vi "Na-DAS_7609 Single.vi"(1 "Single Na-Das Device":T1) -> (0 "DAQ Error":errorcluster)   [LabVIEW 2021]
doc: "Use this plug-in with the Nathan 7609 data acquisition system"
uses:
  Device ID port info.ctl
  Sub_vis/Upload Data.ctl
  Globals/Meas_global.vi
  Globals/Extra_Commands_Global.vi
  Globals/Trav_pos_global.vi
  Globals/Dynamic_call_global.ph.vi
panel:
  in  "Minimum timeout (ms)":u32=15000
  in  "Input voltage range (V)":u8(ring)=1 items=["-5... +5 V", "-10... +10 V"]
  out "Config read-back ok":bool
  out "Overruns":u32
  # "Do not close this window between blocks"
  # "PN 25/11/2014, 19/12/2014, 15/02/2015 (channels in any order), 17/08/2015 (stop ack mod), 23/08/2015 (timeout mod for SW vs HW triggering), 03/09/2017 (rising and falling edge options for HW triggering), 06/06/2018 (rendezvous),"
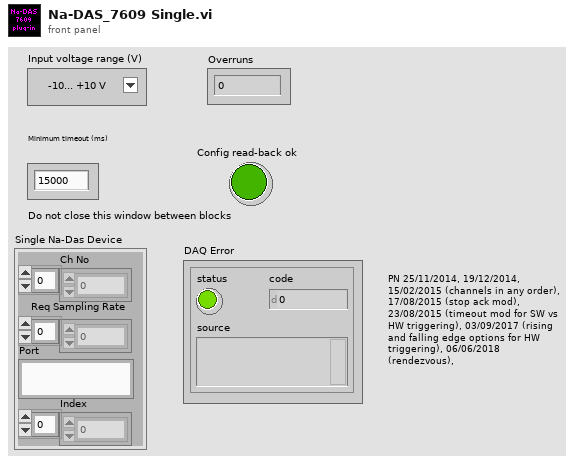
[diagram p1: front panel]
types:
  T1 = typedef "Device ID port info.ctl" = cluster{"Ch No":i16[], "Req Sampling Rate":dbl[], "Port":string, "Index":i32[]}
  T2 = typedef "Traverse_cluster.ctl" = cluster{"Start X":sgl, "Start Y":sgl, "Start Z":sgl, "End X":sgl, "End Y":sgl, "End Z":sgl, "nPoints":i32, "Spacing":T3, "Filename":path, "Tunnel Speed":dbl, "Averaging time (mins)":dbl, "Extra Commands":string, "Carrier_1 Q (l/min)":dbl, "Carrier_2 Q (l/min)":dbl, "Trace Gas Concentration (%)":dbl, "Specific Arguments":string, "Comments":string, "Row No":i32, "Row Type Selector":T4, "EstCompl":string, "Row Duration (mins)":dbl, "nValidPoints":i32, "Meas Setup File":string}
  T3 = typedef "Spacing.ctl" = enum16{"Linear", "Log", "Gauss", "Specified", "N/A"}
  T4 = typedef "Multi_run_mode.ctl" = enum16{"Move Traverse Only", "Set Tunnel Speed Only", "Set Source Only", "Set Measurement Conditions", "Single Measurement", "Vertical Profile", "Lateral Profile", "Longitudinal Profile", "Multi-Axis Profile", "Explore Volume", "Auto Calibrate", "Meas Fast FID Bkgnd", "Check Beam Power", "Scanning Valve Measurement", "Run VI Named:", "Set ADAM Ch", "Wait (minutes)", "Send Message", "Synchronize With:", "Fall Back to this Row", "Turn Off Row Repeating", "Traverse 3D Volume", "Blank Row", "Jump to Fall Back Row"}
  T5 = typedef "Trigger_Mode.ctl" = enum16{"Free Running", "Start on Trigger", "Trigger Every Block", "Trigger Every Sample"}
  T6 = typedef "Setup.ctl" = enum16{"Run Program", "Show Setup", "Save Current Setup", "Setup Front Panel"}
  T7 = typedef "Upload Data.ctl" = enum16{"Voltage Array", "Time Trace Cluster"}
  T8 = typedef "NA-Das_7609.ctl" = cluster{"Timeout (ms)":u32, "N channels bytes to read":u8, "Triggering mode":u8, "Input voltage range (V)":u8, "Oversampling ratio":u8}
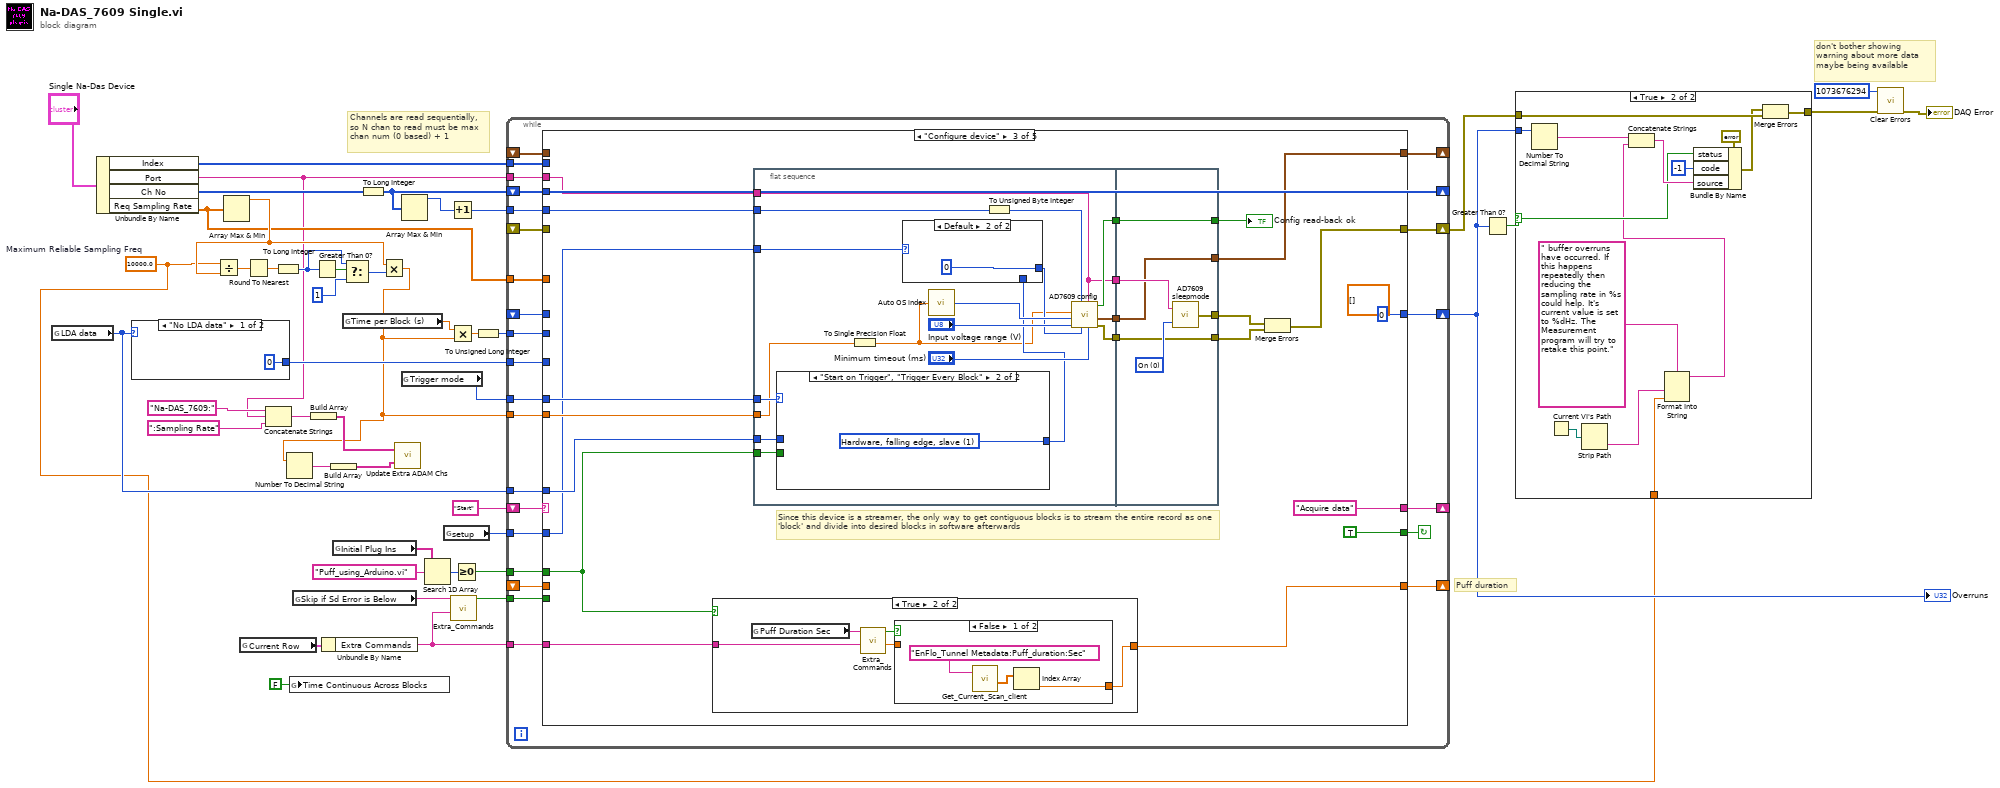
[diagram p0: block diagram]
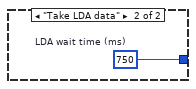
[diagram p3: hidden frame]
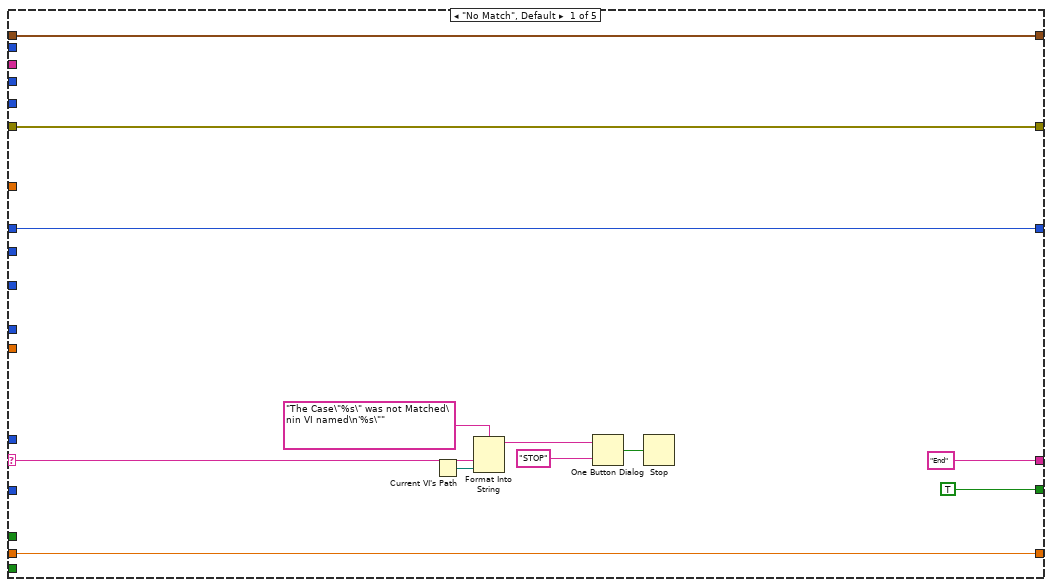
[diagram p4: hidden frame]
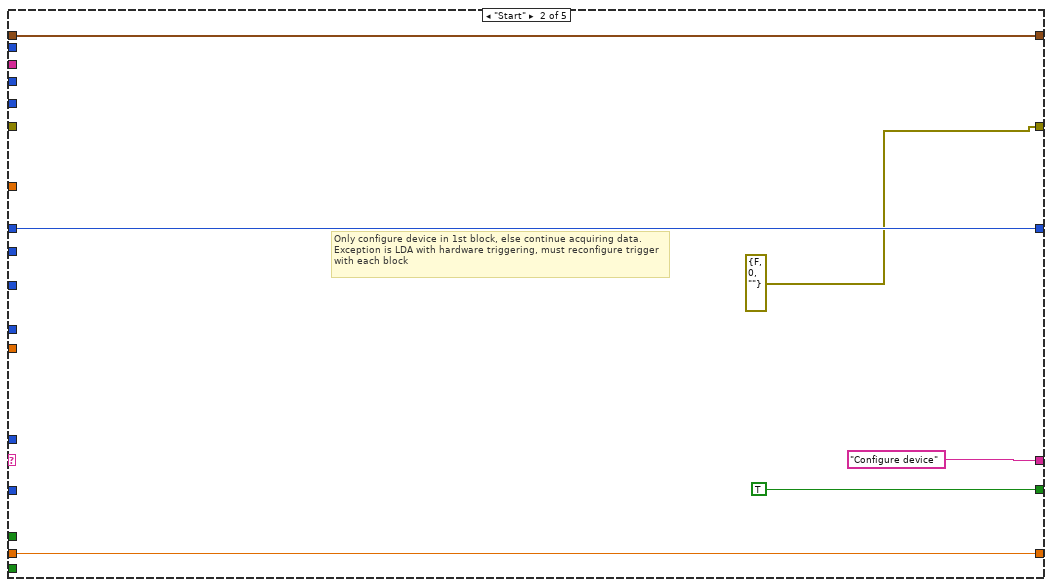
[diagram p5: hidden frame]
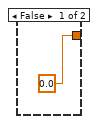
[diagram p6: hidden frame]
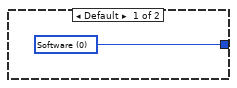
[diagram p9: hidden frame]
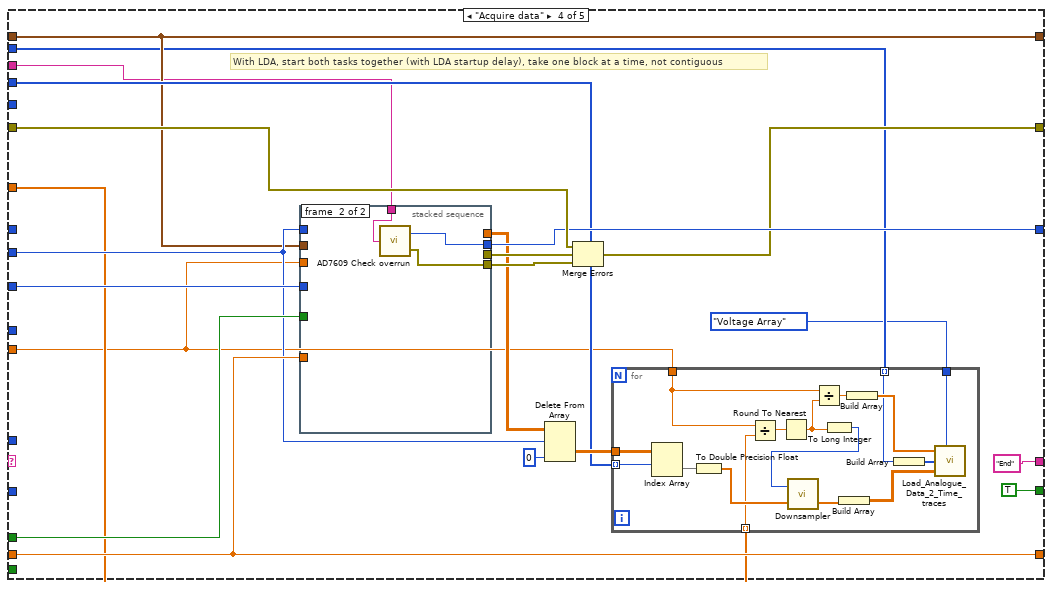
[diagram p10: hidden frame]
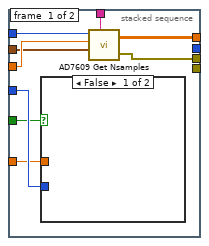
[diagram p11: hidden frame]
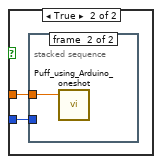
[diagram p12: hidden frame]
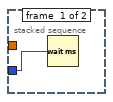
[diagram p13: hidden frame]
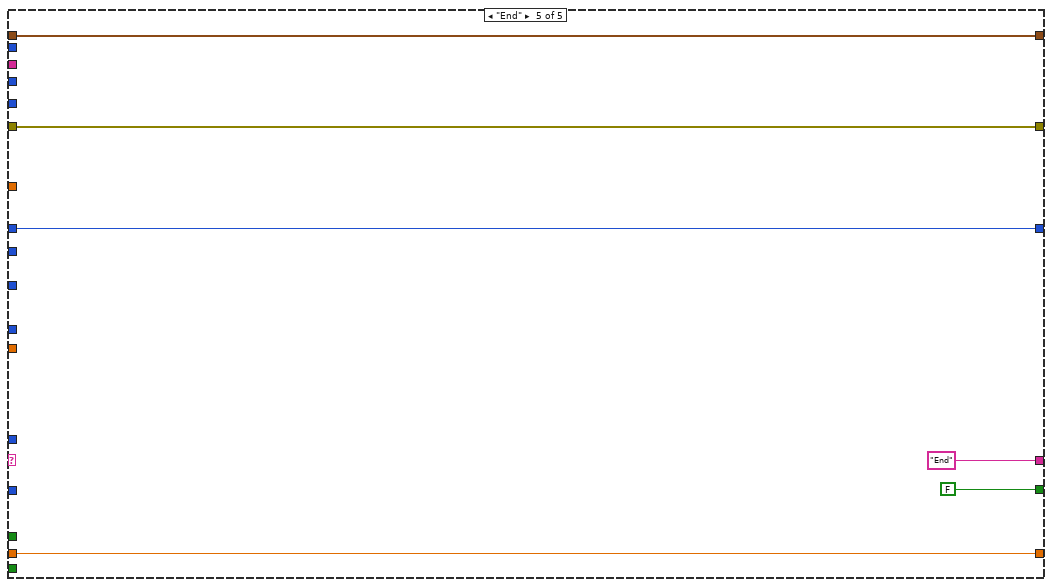
[diagram p14: hidden frame]
diagram:
  w1 = 10000.0  # Maximum Reliable Sampling Freq
  # "don't bother showing warning about more data maybe being available"
  # "Puff duration"
  # "Channels are read sequentially, so N chan to read must be max chan num (0 based) + 1"
  n1 = global read "Meas_global.vi" "LDA data"() -> (w44:enum16{"No LDA data", "Take LDA data"})
  n2 = Unbundle By Name("Single Na-Das Device") -> ("Index"=w22:i32[], "Port"=w8:string, "Ch No"=w21:i16[], "Req Sampling Rate"=w14:dbl[])
  n3 = case shown="\"No LDA data\"" w44 {
    tunnel: [u32 0 ("LDA wait time (ms)") w48] -> w39
    frame "No LDA data" {
    }
    frame "Take LDA data" {
      w48 = u32 750  # LDA wait time (ms)
    }
  }
  n4 = Array Max & Min(array=w14) -> (max value=w15:dbl)  [unwired: 3 out]
  n5 = Divide(x=w1, y=w15) -> (x/y=w17:dbl)
  n6 = global read "Trav_pos_global.vi" "Current Row"() -> (w32:T2)
  n7 = Round To Nearest(number=w17) -> (nearest integer value=w16:dbl)
  n8 = Concatenate Strings("Na-DAS_7609:", w8, ":Sampling Rate") -> (w6:string)
  n9 = To Long Integer(number=w16) -> (32bit integer=w12:i32)
  n10 = global write "Meas_global.vi" "Time Continuous Across Blocks"(FALSE ("Time Continuous Across Blocks")) -> ()
  n11 = global read "Extra_Commands_Global.vi" "Skip if Sd Error is Below"() -> (w31:string)
  n12 = Build Array(w6) -> (w4:string[])
  n13 = Greater Than 0?(x=w12) -> (x > 0?=w13:bool)
  n14 = Unbundle By Name(w32) -> ("Extra Commands"=w30:string)
  n15 = global read "Dynamic_call_global.ph.vi" "Initial Plug Ins"() -> (w41:string[])
  n16 = global read "Meas_global.vi" "Time per Block (s)"() -> (w24:dbl)
  n17 = Select(t=w12, s=w13, f=1) -> (s? t:f=w10:i32)
  n18 = To Long Integer(number=w21) -> (32bit integer=w35:i32[])
  n19 = Multiply(x=w15, y=w10) -> (x*y=w2:dbl)
  n20 = Number To Decimal String(number=w2) -> (decimal integer string=w5:string)  [unwired: 1 in]
  n21 = Build Array(w5) -> (w3:string[])
  n22 = call "Update Extra ADAM Chs.vi"("Extra Ch Values"=w3, "Extra Ch Names"=w4) -> ()  [unwired: 2 in]
  n23 = Array Max & Min(array=w35) -> (max value=w34:i32)  [unwired: 3 out]
  n24 = global read "Meas_global.vi" "Trigger mode"() -> (w45:T5)
  n25 = Search 1D Array(1D array=w41, element="Puff_using_Arduino.vi") -> (index of element=w43:i32)  [unwired: 1 in]
  n26 = global read "Meas_global.vi" "setup"() -> (w20:T6)
  n27 = Increment(x=w34) -> (x+1=w33:i32)
  n28 = Multiply(x=w24, y=w2) -> (x*y=w23:dbl)
  n29 = call "Extra_Commands.vi"("String to Search"=w30, "Command"=w31) -> ("Command Found"=w29:bool)  [unwired: 2 in, 3 out]
  n30 = Greater Or Equal To 0?(x=w43) -> (x >= 0?=w40:bool)
  n31 = To Unsigned Long Integer(number=w23) -> (unsigned 32bit integer=w36:u32)
  n32 = while {
    shift-left: "Start" -> [w73]
    shift-right: [w63] -> _
    tunnel: w2 -> [w72]
    tunnel: w36 -> [w71]
    tunnel: w45 -> [w69]
    tunnel: w44 -> [w68]
    shift-right: [w66] -> w38
    shift-left: _ -> [w67]
    shift-right: [w65] -> w27
    shift-left: _ -> [w64]
    tunnel: w39 -> [w62]
    tunnel: w40 -> [w61]
    shift-right: [w60] -> _
    shift-left: _ -> [w59]
    shift-right: [w58] -> _
    shift-left: w35 -> [w58]
    tunnel: w33 -> [w57]
    tunnel: w30 -> [w56]
    tunnel: w29 -> [w55]
    tunnel: w8 -> [w54]
    tunnel: w22 -> [w53]
    tunnel: w20 -> [w52]
    shift-right: [w51] -> _
    shift-left: _ -> [w50]
    tunnel: w14 -> [w49]
    stop <- w70 continue-if-true
    n33 = case shown="\"Configure device\"" w73 {
      selector: w73 -> [w78 _ _ _ _]
      tunnel: ["End" "Configure device" ("f") "Acquire data" ("f") "End" "End" ("f")] -> w63
      tunnel: w72 -> [_ _ w103 w152 _]
      tunnel: w71 -> [_ _ _ w156 _]
      tunnel: [TRUE TRUE TRUE TRUE FALSE] -> w70
      tunnel: w69 -> [_ _ w102 _ _]
      tunnel: w68 -> [_ _ w97 _ _]
      tunnel: w67 -> [w77 _ _ w168 w206]
      tunnel: [w77 errorcluster {"status"=FALSE, "code"=0, "source"=""} ("error out") w111 w162 w206] -> w66
      tunnel: [w76 w90 u32 0 ("Overruns") w167 w205] -> w65
      tunnel: w64 -> [w76 w90 _ _ w205]
      tunnel: w62 -> [_ _ _ w166 _]
      tunnel: w61 -> [_ _ w96 w165 _]
      tunnel: [w75 w89 w101 w164 w204] -> w60
      tunnel: w59 -> [w75 w89 _ w164 w204]
      tunnel: w58 -> [_ _ _ w161 _]
      tunnel: w57 -> [_ _ w100 _ _]
      tunnel: w56 -> [_ _ w99 _ _]
      tunnel: w55 -> [_ _ _ _ _]
      tunnel: w54 -> [_ _ w98 w154 _]
      tunnel: w53 -> [_ _ _ w151 _]
      tunnel: w52 -> [_ _ w95 _ _]
      tunnel: [w74 w86 w93 w155 w203] -> w51
      tunnel: w50 -> [w74 w86 _ w155 w203]
      tunnel: w49 -> [_ _ _ w153 _]
      frame "No Match", Default {
        n34 = Current VI's Path() -> (path=w81:path)
        n35 = Format Into String(format string="The Case\"%s\" was not Matched\nin VI named\n'%s\"" ("Format String"), w78, w81) -> (resulting string=w84:string)  [unwired: 2 in, 1 out]
        n36 = One Button Dialog(message=w84, button name ("OK")="STOP") -> (true=w82:bool)
        n37 = Stop(stop? (T)=w82) -> ()
      }
      frame "Start" {
        # "Only configure device in 1st block, else continue acquiring data. Exception is LDA with hardware triggering, must reconfigure trigger with each block"
      }
      frame "Configure device" {
        (unwired) sgl[][] [] ("Channel volts")
        # "Since this device is a streamer, the only way to get contiguous blocks is to stream the entire record as one 'block' and divide into desired blocks in software afterwards"
        n38 = case shown="True" w96 {
          tunnel: [0.0 w118] -> w101
          tunnel: w99 -> [_ w114]
          frame False {
          }
          frame True {
            n39 = global read "Extra_Commands_Global.vi" "Puff Duration Sec"() -> (w117:string)
            n40 = call "Extra_Commands.vi"("String to Search"=w114, "Command"=w117) -> ("Numeric Value"=w115:dbl, "Command Found"=w116:bool)  [unwired: 2 in, 2 out]
            n41 = case shown="False" w116 {
              tunnel: [w120 w122] -> w118
              tunnel: w115 -> [_ w122]
              frame False {
                n42 = call "Get_Current_Scan_client.vi"("singleChannel"="EnFlo_Tunnel Metadata:Puff_duration:Sec") -> ("Numerical Values"=w121:dbl[])  [unwired: 1 in, 3 out]
                n43 = Index Array(array=w121) -> (element=w120:dbl)  [unwired: 1 in]
              }
              frame True {
              }
            }
          }
        }
        n44 = flat-sequence {
          tunnel: w103 -> [w134]
          tunnel: w102 -> [w139]
          tunnel: [w137] -> w110
          tunnel: [w136] -> w109
          tunnel: w100 -> [w132]
          tunnel: w98 -> [w124]
          tunnel: w97 -> [w130]
          tunnel: w96 -> [w129]
          tunnel: w95 -> [w128]
          tunnel: [w124] -> w94
          tunnel: [w123] -> w92
          tunnel: [w148] -> w106
          tunnel: w110 -> [w148]
          tunnel: [w147] -> w108
          tunnel: w109 -> [w147]
          tunnel: [w146] -> w107
          tunnel: w94 -> [w145]
          tunnel: [w144] -> w93
          tunnel: w92 -> [w144]
          frame #0 {
            n45 = case shown="\"Start on Trigger\", \"Trigger Every Block\"" w139 {
              tunnel: [w142 w143] -> w126
              tunnel: w130 -> [_ _]
              tunnel: w129 -> [_ _]
              frame Default {
                w142 = u8 0 items=["Software", "Hardware, falling edge, slave", "Hardware, rising edge, slave", "Hardware, falling edge, master", "Hardware, rising edge, master"] ("Triggering mode")
              }
              frame "Start on Trigger", "Trigger Every Block" {
                w143 = u8 1 items=["Software", "Hardware, falling edge, slave", "Hardware, rising edge, slave", "Hardware, falling edge, master", "Hardware, rising edge, master"] ("Triggering mode")
              }
            }
            n46 = To Single Precision Float(number=w134) -> (single precision float=w125:sgl)
            n47 = case shown="Default" w128 {
              tunnel: [w140 u8 0 ("Triggering mode")] -> w127
              tunnel: w126 -> [w140 _]
              frame "Run Program" {
              }
              frame Default {
              }
            }
            n48 = call "Auto OS index.vi"("Sampling rate"=w125) -> ("OS index"=w133:u8)
            n49 = To Unsigned Byte Integer(number=w132) -> (unsigned 8bit integer=w138:u8)
            n50 = call "AD7609 config.vi"("Timeout for software trig. mode (ms)"="Minimum timeout (ms)", "Device serial port"=w124, "Triggering mode"=w127, "N channels to read"=w138, "Input voltage range (V)"="Input voltage range (V)", "Oversampling ratio"=w133, "Sampling rate (Hz)"=w125) -> ("Config error out"=w136:errorcluster, "Device Parameters"=w123:T8, "Config read-back ok"=w137:bool)  [unwired: 2 in]
          }
          frame #1 {
            w149 = u8 0 items=["On", "Standby", "Shutdown"] ("Sleep state")
            n51 = call "AD7609 sleepmode.vi"("Sleep state"=w149, "VISA resource name"=w145) -> ("Sleep error out"=w146:errorcluster)
          }
        }
        n52 = Merge Errors(w107, w108) -> (w111:errorcluster)
        "Config read-back ok" <- w106
      }
      frame "Acquire data" {
        # "With LDA, start both tasks together (with LDA startup delay), take one block at a time, not contiguous"
        n53 = stacked-sequence {
          tunnel: [_ w186] -> w167
          tunnel: [w176 _] -> w157
          tunnel: [w175 _] -> w160
          tunnel: w166 -> [w179 _]
          tunnel: w165 -> [w178 _]
          tunnel: w164 -> [w177 _]
          tunnel: [_ w185] -> w158
          tunnel: w156 -> [w174 _]
          tunnel: w152 -> [w173 _]
          tunnel: w155 -> [w172 _]
          tunnel: w154 -> [w171 w184]
          frame #0 {
            n54 = case shown="False" w178 {
              tunnel: w177 -> [_ w181]
              tunnel: w179 -> [_ w180]
              frame False {
              }
              frame True {
                n55 = stacked-sequence {
                  tunnel: w181 -> [_ w183]
                  tunnel: w180 -> [w182 _]
                  frame #0 {
                    n56 = Wait (ms)(milliseconds to wait=w182) -> ()  [unwired: 1 out]
                  }
                  frame #1 {
                    n57 = call "Puff_using_Arduino_oneshot.vi"("Puff_duration:Sec"=w183) -> ()  [unwired: 7 in]
                  }
                }
              }
            }
            n58 = call "AD7609 Get Nsamples.vi"("Number of Samples"=w174, "Sampling Rate (Hz)"=w173, "Device Parameters"=w172, "VISA resource name"=w171) -> ("Channel volts"=w176:sgl[][], "Error out"=w175:errorcluster)  [unwired: 1 in]
          }
          frame #1 {
            n59 = call "AD7609 Check overrun.vi"("VISA resource name"=w184) -> ("Overruns"=w186:u32, "Overrun error out"=w185:errorcluster)
          }
        }
        n60 = Delete From Array(array=w157, length=w156, index (col)=0 ("disabled index (col)")) -> (deleted portion=w163:sgl[][])  [unwired: 1 in, 1 out]
        n61 = Merge Errors(w168, w160, w158) -> (w162:errorcluster)
        n62 = for {
          tunnel: w161 -> [w201] mode=indexing
          tunnel: w163 -> [w202]
          tunnel: w153 -> [w198] mode=indexing
          tunnel: w152 -> [w194]
          tunnel: w151 -> [w188] mode=indexing
          tunnel: Upload_Data."Voltage Array" ("Mode") -> [w191]
          n63 = Index Array(array=w202, index (row)=w201) -> (element=w200:sgl[])  [unwired: 1 in]
          n64 = To Double Precision Float(number=w200) -> (double precision float=w199:dbl[])
          n65 = Divide(x=w194, y=w198) -> (x/y=w197:dbl)
          n66 = Round To Nearest(number=w197) -> (nearest integer value=w195:dbl)
          n67 = Divide(x=w194, y=w195) -> (x/y=w190:dbl)
          n68 = To Long Integer(number=w195) -> (32bit integer=w196:i32)
          n69 = call "Downsampler.vi"("Input Array"=w199, "Averaging samples"=w196) -> ("Downsampled Array"=w193:dbl[])  [unwired: 1 out]
          n70 = Build Array(w193) -> (w192:dbl[][])
          n71 = Build Array(w190) -> (w189:dbl[])
          n72 = Build Array(w188) -> (w187:i32[])
          n73 = call "Load_Analogue_Data_2_Time_traces.vi"("Sampling Rate (Hz)"=w189, "Mode"=w191, "Index"=w187, "Voltage Array"=w192) -> ()  [unwired: 3 in]
        }
      }
      frame "End" {
      }
    }
  }
  "Overruns" <- w27
  n74 = Greater Than 0?(x=w27) -> (x > 0?=w28:bool)
  n75 = case shown="True" w28 {
    selector: w28 -> [_ w216]
    tunnel: w38 -> [w209 w222]
    tunnel: [w209 w223] -> w37
    tunnel: w27 -> [_ w221]
    tunnel: w1 -> [_ w210]
    frame False {
    }
    frame True {
      n76 = Number To Decimal String(number=w221) -> (decimal integer string=w220:string)  [unwired: 1 in]
      n77 = Current VI's Path() -> (path=w213:path)
      n78 = Strip Path(path=w213) -> (name=w211:string)  [unwired: 1 out]
      n79 = Format Into String(format string=" buffer overruns have occurred. If this happens repeatedly then reducing the sampling rate in %s could help. It's current value is set to %dHz. The Measurement program will try to retake this point.", w211, w210) -> (resulting string=w212:string)  [unwired: 2 in, 1 out]
      n80 = Concatenate Strings(w220, w212) -> (w218:string)
      n81 = Bundle By Name(cluster=errorcluster {"status"=FALSE, "code"=0, "source"=""} ("error IO"), "status"=w216, "code"=-1, "source"=w218) -> (w215:errorcluster)
      n82 = Merge Errors(w215, w222) -> (w223:errorcluster)
    }
  }
  n83 = call <vilib>:"Clear Errors.vi"("error in (no error)"=w37, "specific error code to clear (0: all)"=1073676294) -> ("error out"=→"DAQ Error":errorcluster)  [unwired: 4 in, 1 out]
